vi "Actor Core.vi"(8 "error in":errorcluster, 11 "Composite User Interface in":refnum<class "Composite User Interface.lvclass">) -> (0 "error out":errorcluster, 3 "Actor out":refnum<class "Actor.lvclass">)   [LabVIEW 2020, in "2. Basic Panel Actors.lvlib" / "Composite User Interface.lvclass"]
doc: "The user interface for this panel.\n----\nCopyright: MGI 2016\nAuthor: Derek Trepanier"
uses:
  Composite User Interface.lvclass
  C:/Program Files/National Instruments/LabVIEW 2020/vi.lib/MGI/Panel Manager/Panel Actor/Panel Actor/Panel Actor.lvclass
  <vilib>/ActorFramework/Actor/Actor.lvclass
  Data Manager/Data Manager.lvclass
  Data Viewer/Data Viewer.lvclass
  <vilib>/ActorFramework/Message Enqueuer/Message Enqueuer.lvclass/Message Enqueuer.ctl
  <vilib>/ActorFramework/Message Enqueuer/Enqueue.vi
  Description Panel/Description Panel.lvclass
  <vilib>/MGI/Panel Manager/Panel/Panel/Subpanel/Subpanel.lvclass
  C:/Program Files/National Instruments/LabVIEW 2020/vi.lib/MGI/Panel Manager/Panel/Panel/Panel.lvclass
  <vilib>/ActorFramework/Stop Msg/Stop Msg.lvclass
  C:/Program Files/National Instruments/LabVIEW 2020/vi.lib/ActorFramework/Message/Message.lvclass
  <vilib>/MGI/Panel Manager/Panel/Panel/Subpanel/Subpanel.vi
  <vilib>/ActorFramework/Message Priority Queue/Priority Enqueue.vi
  <vilib>/MGI/Panel Manager/Panel Actor/Panel Actor/Panel Actor.lvclass
  <vilib>/MGI/Panel Manager/Panel/Panel.lvlib
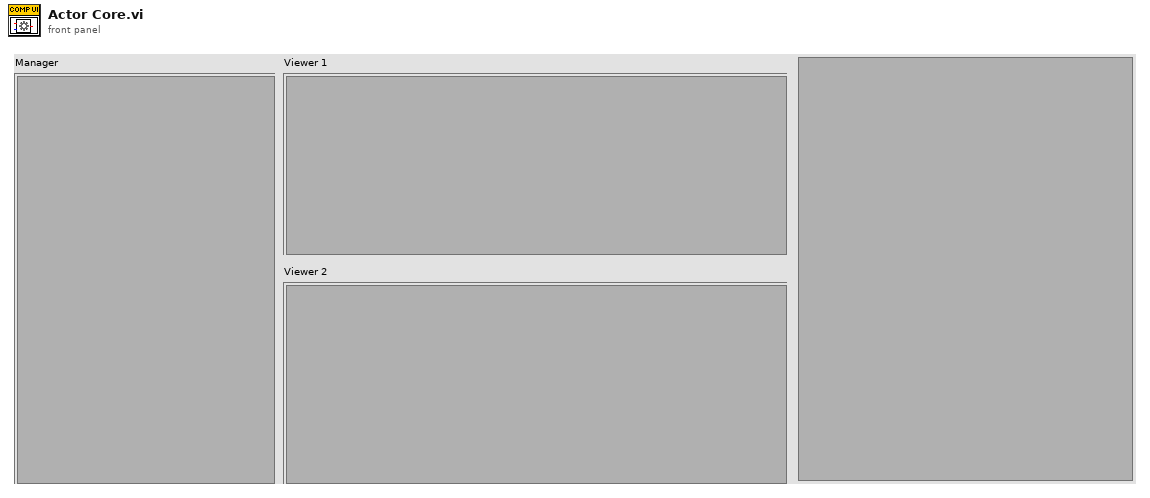
[diagram p1: front panel]
types:
  T1 = cluster{"2. Basic Panel Actors.lvlib:Data Viewer.lvclass":refnum<class "Data Viewer.lvclass">, "Subpanel Out":refnum<class "Subpanel.lvclass">}
  T2 = cluster{"Description Panel out":refnum<class "Description Panel.lvclass">, "Subpanel Out":refnum<class "Subpanel.lvclass">}
  T3 = cluster{"2. Basic Panel Actors.lvlib:Data Manager.lvclass":refnum<class "Data Manager.lvclass">, "Subpanel Out":refnum<class "Subpanel.lvclass">}
  T4 = cluster{"2. Basic Panel Actors.lvlib:Data Manager.lvclass":refnum<class "Panel Actor.lvclass">, "Subpanel Out":refnum<class "Subpanel.lvclass">}[]
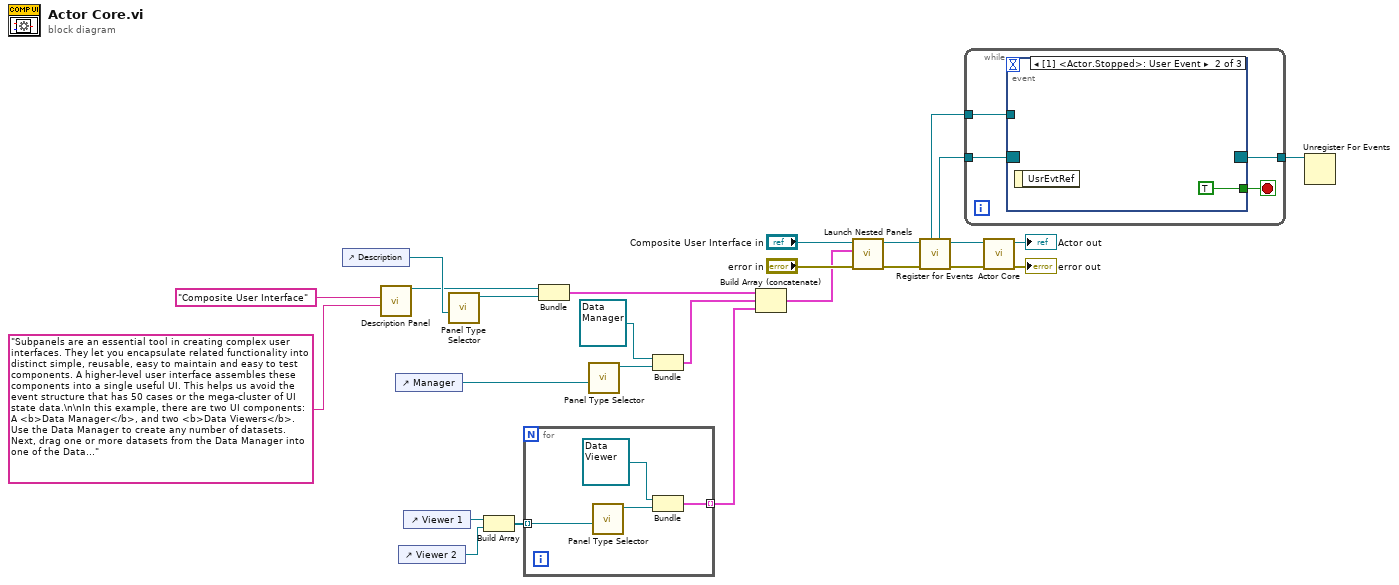
[diagram p0: block diagram]
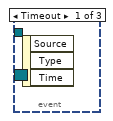
[diagram p2: hidden frame]
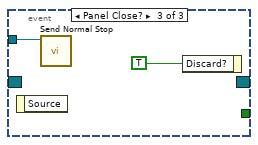
[diagram p3: hidden frame]
diagram:
  n1 = control-ref of="Description"() -> (w20:refnum<vi>)
  n2 = call "Description Panel.vi"("Description"="Subpanels are an essential tool in creating complex user interfaces. They let you encapsulate related functionality into distinct simple, reusable, easy to maintain and easy to test components. A higher-level user interface assembles these components into a single useful UI. This helps us avoid the event structure that has 50 cases or the mega-cluster of UI state data.\n\nIn this example, there are two UI components: A <b>Data Manager</b>, and two <b>Data Viewers</b>. Use the Data Manager to create any number of datasets. Next, drag one or more datasets from the Data Manager into one of the Data Viewers. \n\nNotice how the top-level UI is trivial. All it does is launch the components and manage closing the application. We also get some nice re-use with Data Viewer component by launching two of the same component in different subpanels on the top-level UI and by being able to launch a Dataset Viewer in a separate window from the Dataset Manager. \n" ("Description Title"), "Description Title"="Composite User Interface") -> ("Description Panel out"=w7:refnum<class "Description Panel.lvclass">)  [unwired: 8 in, 1 out]
  n3 = control-ref of="Manager"() -> (w17:refnum<vi>)
  n4 = control-ref of="Viewer 2"() -> (w15:refnum<vi>)
  n5 = control-ref of="Viewer 1"() -> (w16:refnum<vi>)
  n6 = call-poly <vilib>:"Panel Type Selector.vi"("Sub Panel"=w20) -> ("Subpanel Out"=w4:refnum<class "Subpanel.lvclass">)  [unwired: 9 in, 1 out]
  n7 = Build Array(w16, w15) -> (w14:refnum<vi>[])
  n8 = for {
    tunnel: w14 -> [w30] mode=indexing
    tunnel: [w27] -> w3 mode=indexing
    n9 = call-poly <vilib>:"Panel Type Selector.vi"("Sub Panel"=w30) -> ("Subpanel Out"=w29:refnum<class "Subpanel.lvclass">)  [unwired: 9 in, 1 out]
    n10 = Bundle("2. Basic Panel Actors.lvlib:Data Viewer.lvclass"=refnum<class "Data Viewer.lvclass"> refnum, "Subpanel Out"=w29) -> (w27:T1)  [unwired: 1 in]
  }
  n11 = Bundle("Description Panel out"=w7, "Subpanel Out"=w4) -> (w6:T2)  [unwired: 1 in]
  n12 = call-poly <vilib>:"Panel Type Selector.vi"("Sub Panel"=w17) -> ("Subpanel Out"=w9:refnum<class "Subpanel.lvclass">)  [unwired: 9 in, 1 out]
  n13 = Bundle("2. Basic Panel Actors.lvlib:Data Manager.lvclass"=refnum<class "Data Manager.lvclass"> refnum, "Subpanel Out"=w9) -> (w5:T3)  [unwired: 1 in]
  n14 = Build Array (concatenate)(w6, w5, w3) -> (w1:T4)
  n15 = call <vilib>:"Launch Nested Panels.vi"("error in (no error)"="error in", "Nested Panel Actors"=w1, "Panel Actor in"="Composite User Interface in") -> ("error out"=w12:errorcluster, "Panel Actor out"=w11:refnum<class "Composite User Interface.lvclass">)  [unwired: 5 in, 2 out]
  n16 = call <vilib>:"Register for Events.vi"("Error In"=w12, "Panel Actor in"=w11) -> ("Error Out"=w22:errorcluster, "Panel Actor out"=w21:refnum<class "Composite User Interface.lvclass">, "Pnl Actor"=w19:refnum<event-registration>, "Self Enqueuer"=w18:refnum<class "Message Enqueuer.lvclass">)  [unwired: 6 in]
  n17 = while {
    tunnel: w19 -> [w34]
    tunnel: w18 -> [w33]
    tunnel: [w31] -> w13
    stop <- w32 stop-if-true
    n18 = event shown="[1] <Actor.Stopped>: User Event" {
      selector: w34 -> [_ _ _]
      dyn-events: [_ _ _] -> w31
      timeout: _ -> [_ _ _]
      tunnel: w33 -> [_ _ w37]
      tunnel: [_ TRUE _] -> w32
      event Timeout {
        n19 = event-data() -> ()  [unwired: 1 in, 3 out]
      }
      event User Event {
        n20 = event-data() -> ()  [unwired: 1 in, 1 out]
      }
      event Panel Close? {
        n21 = event-data() -> ()  [unwired: 1 in, 1 out]
        n22 = call <vilib>:"Send Normal Stop.vi"("Message Enqueuer"=w37) -> ()  [unwired: 10 in, 1 out]
        n23 = event-data("Discard?"=TRUE) -> ()  [unwired: 1 in, 1 out]
      }
    }
  }
  n24 = call-parent "Actor Core.vi"("error in"=w22, "Panel Actor in"=w21) -> ("error out"=→"error out":errorcluster, "Actor out"=→"Actor out":refnum<class "Actor.lvclass">)  [unwired: 8 in]
  n25 = Unregister For Events(event registration refnum=w13) -> ()  [unwired: 1 in, 1 out]
